vi "Boolean Test.vi"() -> ()   [LabVIEW 2013]
panel:
  out "Boolean 2":bool
  in  "stop":bool
  in  "OK Button":bool
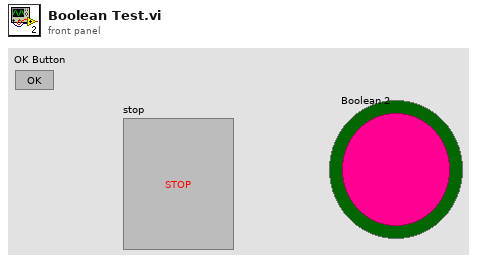
[diagram p1: front panel]
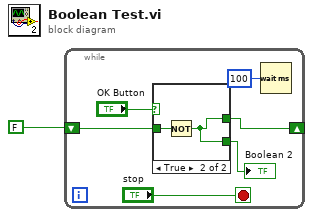
[diagram p0: block diagram]
diagram:
  n1 = while {
    shift-right: [w6] -> _
    shift-left: FALSE -> [w7]
    stop <- "stop" stop-if-true
    n2 = case shown="True" "OK Button" {
      tunnel: [w8 w9] -> w6
      tunnel: w7 -> [w8 w10]
      tunnel: [w8 w9] -> w3
      frame False {
      }
      frame True {
        n3 = Not(x=w10) -> (.not. x?=w9:bool)
      }
    }
    "Boolean 2" <- w3
    n4 = Wait (ms)(milliseconds to wait=u32 100) -> ()  [unwired: 1 out]
  }
